vi "MeasureWhileChanging.vi"(8 "error in (no error)":errorcluster, 11 "AcPwrBase in":refnum<class "AcPwrBase.lvclass">) -> (0 "error out":errorcluster, 1 "MeasureWhileChangingConfigurationSettings":bool, 2 "MeasureWhileChangingOutput/LoadState":bool, 3 "AcPwrBase Out":refnum<class "AcPwrBase.lvclass">)   [LabVIEW 2018, in "AcPwrPlugins.lvlib" / "AcPwrBase.lvclass"]
doc: "This VI retrieves a boolean status to see if the instrument can conduct measurements while the device is changing modes or turning off and on."
uses:
  AcPwrBase.lvclass
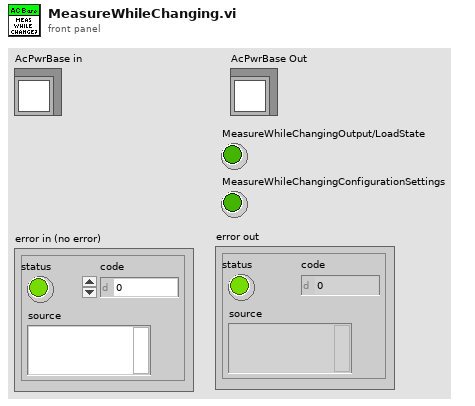
[diagram p1: front panel]
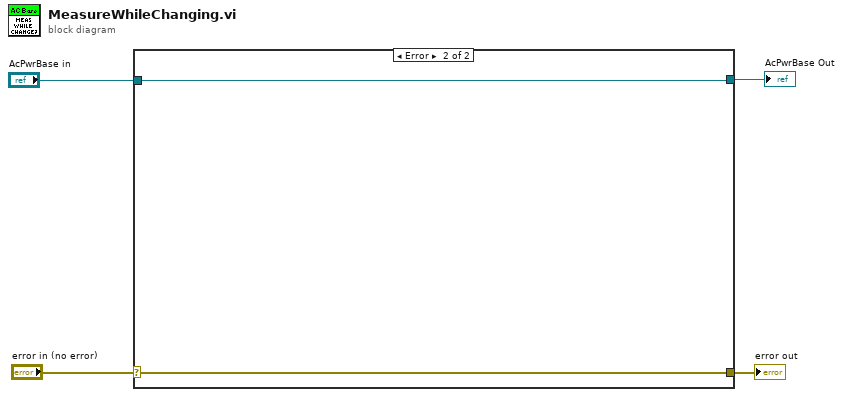
[diagram p0: block diagram]
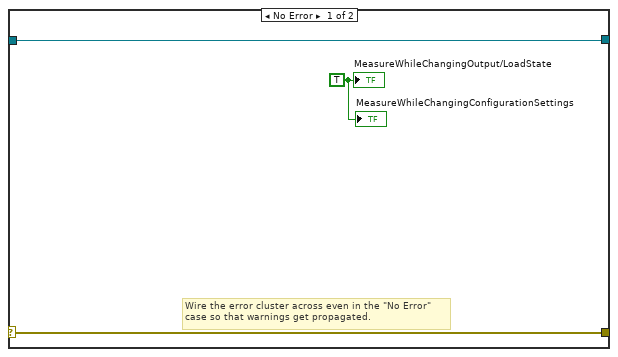
[diagram p2: hidden frame]
diagram:
  n1 = case shown="Error" "error in (no error)" {
    selector: "error in (no error)" -> [w7 w9]
    tunnel: [w7 w9] -> w3
    tunnel: "AcPwrBase in" -> [w5 w8]
    tunnel: [w5 w8] -> w1
    frame No Error {
      w6 = TRUE ("MeasureWhileChangingOutput/LoadValues")
      # "Wire the error cluster across even in the \"No Error\"\ncase so that warnings get propagated."
      "MeasureWhileChangingOutput/LoadState" <- w6
      "MeasureWhileChangingConfigurationSettings" <- w6
    }
    frame Error {
    }
  }
  "error out" <- w3
  "AcPwrBase Out" <- w1
